vi "Set_ReadoutControlMode.vi"(8 "error in":errorcluster, 10 "ReadoutControlMode":T1=1 items=["FullFrame"=1, "FrameTransfer"=2, "Kinetics"=3, "SpectraKinetics"=4, "Interline"=5, "Dif"=6, "SeNsR"=7, "RollingShutter"=8], 11 "camera handle in":u64) -> (0 "error out":errorcluster, 3 "camera handle out":u64)   [LabVIEW 2019, in "PICam.lvlib"]
doc: "FullFrame\nThe sensor is read one frame at a time.\n\nFrameTransfer \nThe sensor is reading out a frame while exposing the next frame.\n\nKinetics \nThe sensor rapidly stores multiple frames and then reads those out.\n\nSpectraKinetics \nSame as kinetics, but optimized to capture a larger burst of spectral frames.\n\nDif \nThe Dual Imaging Feature where the sensor acquires two frames rapidly and then reads them both out."
uses:
  PICam.lvlib
  Ctrls/ReadoutControlMode.ctl
  Picam64.dll   
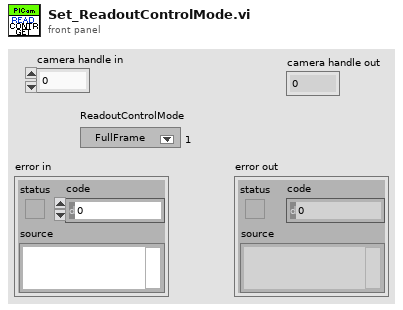
[diagram p1: front panel]
types:
  T1 = typedef "PICam.lvlib/ReadoutControlMode.ctl" = u32
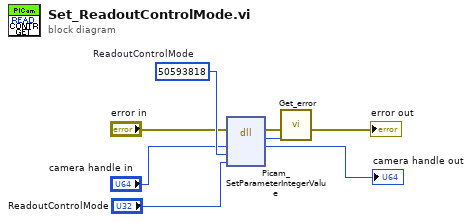
[diagram p0: block diagram]
diagram:
  w4 = u32 50593818  # ReadoutControlMode
  n1 = dll-call lib="Picam32.dll" fn="Picam_SetParameterIntegerValue"(error in="error in", "camera"="camera handle in", "PicamParameter"=w4, "ReadoutControlMode"="ReadoutControlMode") -> (error out=w8:errorcluster, "return type"=w7:i32, "camera"=→"camera handle out":u64)  [unwired: 4 in, 1 out]
  n2 = call "Get_error.vi"("PICam_Error"=w7, "error in (no error)"=w8) -> ("error out"=→"error out":errorcluster)  [unwired: 9 in]
